vi "Set mode DSP402.vi"(4 "error in (no error)":errorcluster, 6 "Mode":T1 items=["Undefined"=0, "Profile Position Mode"=1, "Velocity Mode"=2, "Profile Velocity Mode"=3, "Torque Profile Mode"=4, "Homing Mode"=6, "Interpolated Position Mode"=7], 7 "DSP402 in":refnum<class "DSP402.lvclass">) -> (0 "error out":errorcluster, 3 "DSP402 out":refnum<class "DSP402.lvclass">)   [LabVIEW 2026, in "canopen_.lvlib" / "DSP402.lvclass"]
uses:
  DSP402.lvclass
  DSP402.lvclass/DSP402.ctl
  CANopen/Multiplexor.ctl
  CANopen Master.lvlib
  Download DSP402 (U8).vi
  DriveMode.ctl
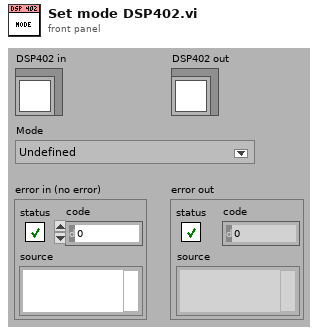
[diagram p1: front panel]
types:
  T1 = typedef "canopen_.lvlib/DSP402.lvclass/DriveMode.ctl" = i8
  T2 = typedef "CANopen Master.lvlib/Multiplexor.ctl" = cluster{"Index":u16, "Sub-Index":i16}
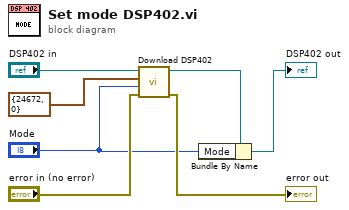
[diagram p0: block diagram]
diagram:
  n1 = call-poly "Download DSP402.vi"("error in (no error)"="error in (no error)", "Value"="Mode", "Multiplexor"=T2 {"Index"=24672, "Sub-Index"=0}, "DSP402 in"="DSP402 in") -> ("error out"=→"error out":errorcluster, "DSP402 out"=w1:refnum<class "DSP402.lvclass">)  [unwired: 2 in]
  n2 = Bundle By Name(cluster=w1, "Mode"="Mode") -> (→"DSP402 out":refnum<class "DSP402.lvclass">)
